vi "hwOperation_Update MeasurementValues.vi"(7 "hwType":string, 8 "Error in":errorcluster, 11 "hwDriverRef in":T1) -> (0 "Error out":errorcluster, 3 "hwDriverRef out":T1)   [LabVIEW 2016]
uses:
  QX/hw_QX_hwDriverRef.ctl
  C:/Users/CL/Desktop/ZcDAQprj0811/ZcDAQprj/Modules/DAQ-Device/Hardware Drivers/QX/HBM LabVIEW Driver/DLLs/Hbm.Api.Common.dll
  QX/HBM LabVIEW Driver/DLLs/Hbm.Api.Common.dll
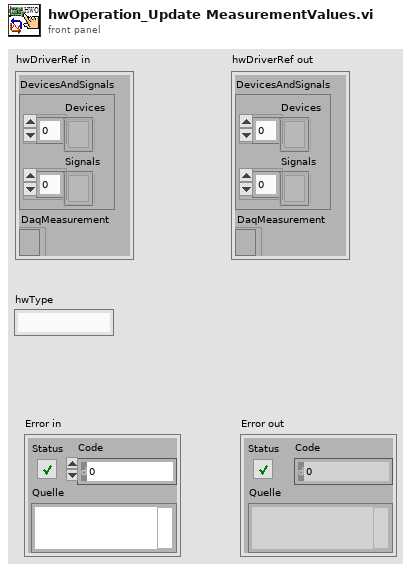
[diagram p1: front panel]
types:
  T1 = typedef "hw_QX_hwDriverRef.ctl" = cluster{"DevicesAndSignals":cluster{"Devices":refnum<k24>[], "Signals":refnum<k24>[]}, "DaqMeasurement":refnum<k24>}
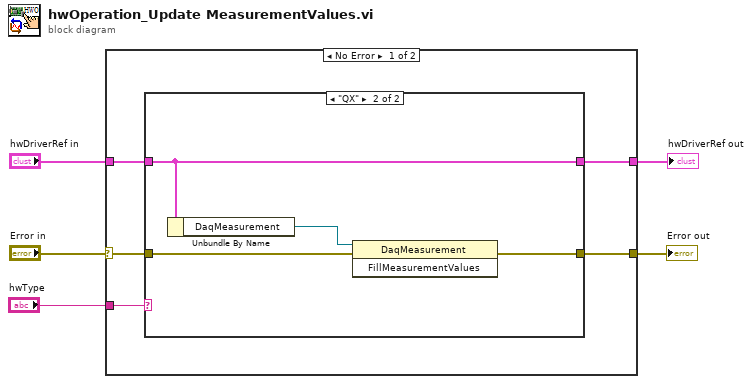
[diagram p0: block diagram]
diagram:
  n1 = case shown="No Error" "Error in" {
    selector: "Error in" -> [w10 w18]
    tunnel: "hwDriverRef in" -> [w6 w17]
    tunnel: [w9 w18] -> w4
    tunnel: [w7 w17] -> w3
    tunnel: "hwType" -> [w8 _]
    frame No Error {
      n2 = case shown="\"QX\"" w8 {
        tunnel: w10 -> [w12 w16]
        tunnel: [w12 w15] -> w9
        tunnel: [w11 w14] -> w7
        tunnel: w6 -> [w11 w14]
        frame "Simulation", Default {
        }
        frame "QX" {
          n3 = Unbundle By Name(w14) -> ("DaqMeasurement"=w13:refnum<k24>)
          n4 = invoke on="Methodenknoten" class="DaqMeasurement" method="FillMeasurementValues"(reference=w13, error in=w16) -> (error out=w15:errorcluster)  [unwired: 1 in, 2 out]
        }
      }
    }
    frame Error {
    }
  }
  "Error out" <- w4
  "hwDriverRef out" <- w3
